vi "BoolSignalChangeCheck.vi"(9 "前回値":bool, 11 "今回値":bool) -> (1 "判定":T1)   [LabVIEW 2014]
uses:
  Ctl/BoolSignalChangeCheck.ctl
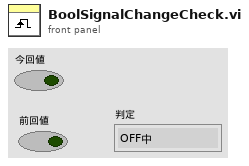
[diagram p1: front panel]
types:
  T1 = typedef "BoolSignalChangeCheck.ctl" = enum16{"OFF中", "立上り", "立下り", "ON中"}
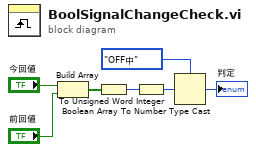
[diagram p0: block diagram]
diagram:
  n1 = Build Array("今回値", "前回値") -> (w6:bool[])
  n2 = Boolean Array To Number(Boolean array=w6) -> (number=w5:u32)
  n3 = To Unsigned Word Integer(number=w5) -> (unsigned 16bit integer=w4:u16)
  n4 = Type Cast(type=BoolSignalChangeCheck."OFF中" ("判定"), x=w4) -> (*(type *) &x=→"判定":T1)
